vi "Mapping Error Dialog (Single).vi"(8 "error in (no error)":errorcluster, 9 "Destination":string, 10 "Source":string, 11 "Error Text":string) -> (0 "error out":errorcluster)   [LabVIEW 2016, in "System Mapping Tool.lvlib"]
uses:
  System Mapping Tool.lvlib
panel:
  in  "OK":bool
  in  "Mapping Errors":i32(listbox)
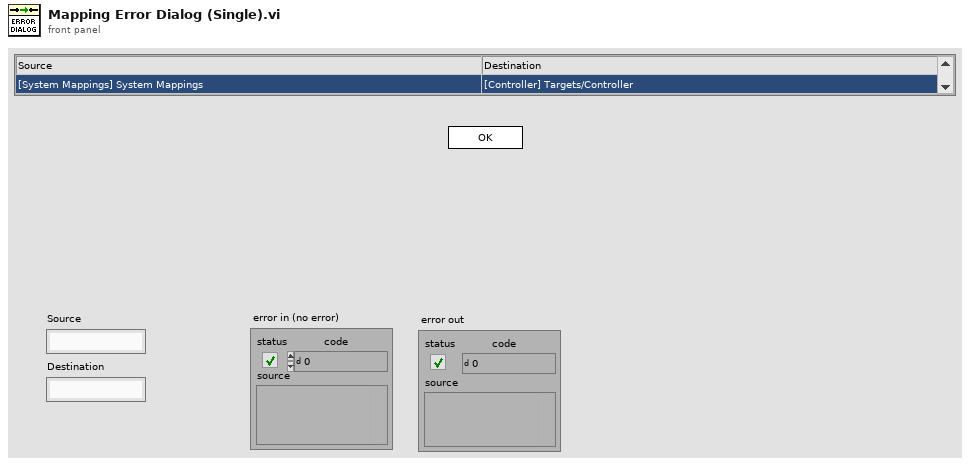
[diagram p1: front panel]
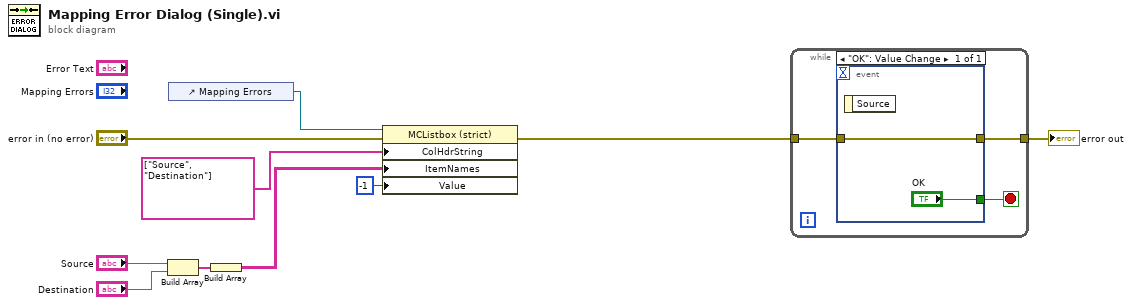
[diagram p0: block diagram]
diagram:
  n1 = Build Array("Source", "Destination") -> (w5:string[])
  n2 = control-ref of="Mapping Errors"() -> (w9:refnum<vi>)
  n3 = Build Array(w5) -> (w4:string[][])
  n4 = property class="MCListbox (strict)"(reference=w9, error in="error in (no error)", "ColHdrString"=string[] ["Source", "Destination"] ("Column Header Strings[]"), "ItemNames"=w4, "Value"=-1) -> (error out=w3:errorcluster)  [unwired: 1 out]
  n5 = while {
    tunnel: [w12] -> w2
    tunnel: w3 -> [w11]
    stop <- w13 stop-if-true
    n6 = event shown="[0] \"OK\": Value Change" {
      selector: _ -> [_]
      dyn-events: _ -> [_]
      timeout: _ -> [_]
      tunnel: ["OK"] -> w13
      tunnel: [w14] -> w12
      tunnel: w11 -> [w14]
      event "OK": Value Change {
        n7 = event-data() -> ()  [unwired: 1 in, 1 out]
      }
    }
  }
  "error out" <- w2
